vi "Send command ADC.vi"(8 "error in (no error)":errorcluster, 9 "Canal":string(combo), 10 "Marca":string, 11 "object in":refnum<class "Simulado.lvclass">) -> (0 "error out":errorcluster, 1 "Expected response":string, 2 "Command":string, 3 "object out":refnum<class "Simulado.lvclass">)   [LabVIEW 2020, in "Simulado.lvclass"]
doc: "Se manda el comando para leer el ADC, se escribe en el puerto serial y se lee la respuesta que de el micro simulado."
uses:
  Simulado.lvclass
  Simulado.lvclass/Simulado.ctl
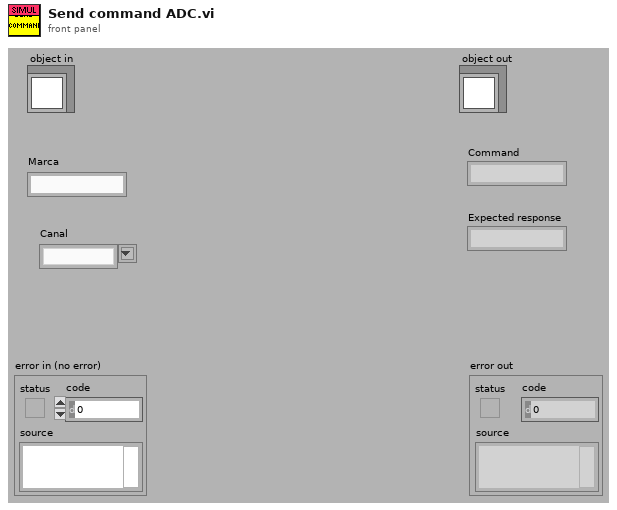
[diagram p1: front panel]
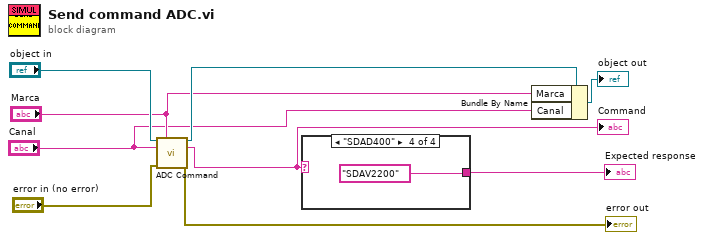
[diagram p0: block diagram]
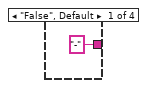
[diagram p2: hidden frame]
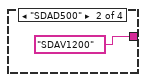
[diagram p3: hidden frame]
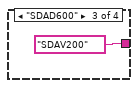
[diagram p4: hidden frame]
diagram:
  n1 = call-dynamic "ADC Command.vi"("object in"="object in", "Marca"="Marca", "Canal"="Canal", "error in (no error)"="error in (no error)") -> ("object out"=w6:refnum<class "Simulado.lvclass">, "Command"=w1:string, "error out"=→"error out":errorcluster)  [unwired: 8 in, 1 out]
  "Command" <- w1
  n2 = case shown="\"SDAD400\"" w1 {
    tunnel: ["-" ("Command") "SDAV1200" ("Command") "SDAV200" ("Command") "SDAV2200" ("Command")] -> w2
    frame "False", Default {
    }
    frame "SDAD500" {
    }
    frame "SDAD600" {
    }
    frame "SDAD400" {
    }
  }
  "Expected response" <- w2
  n3 = Bundle By Name(cluster=w6, "Marca"="Marca", "Canal"="Canal") -> (→"object out":refnum<class "Simulado.lvclass">)
